vi "关键字子集.vi"(8 "图形程序":refnum<vi>, 9 "关键字":refnum<vi>, 10 "结束坐标":T1, 11 "起始坐标":T1) -> (0 "选中子集":cluster{"行":i32, "列":i32}[](array[cluster]))   [LabVIEW 2020]
uses:
  <vilib>/Utility/miscctls.llb/LVPoint32TypeDef.ctl
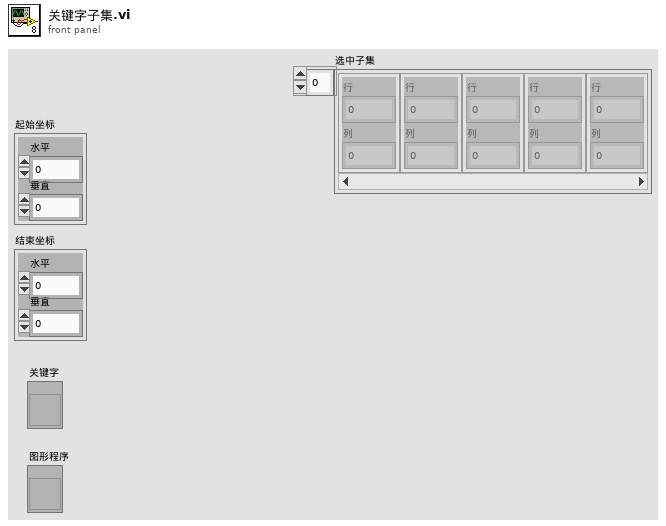
[diagram p1: front panel]
types:
  T1 = typedef "LVPoint32TypeDef.ctl" = cluster{"Horizontal":i32, "Vertical":i32}
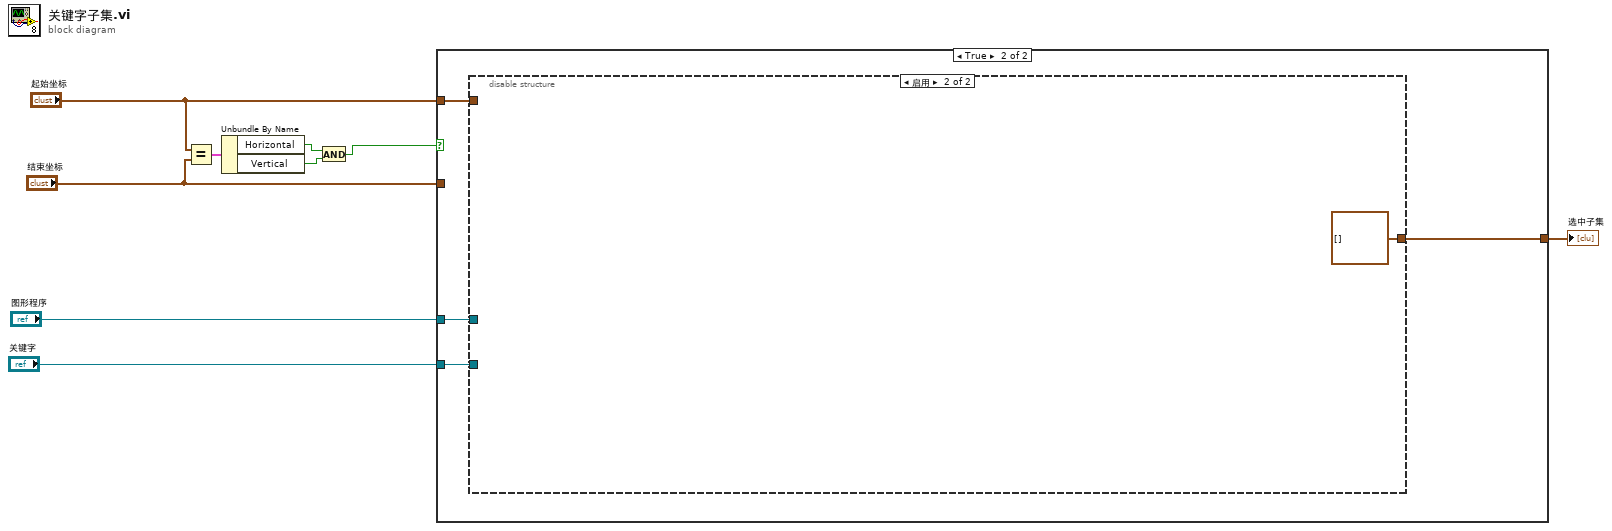
[diagram p0: block diagram]
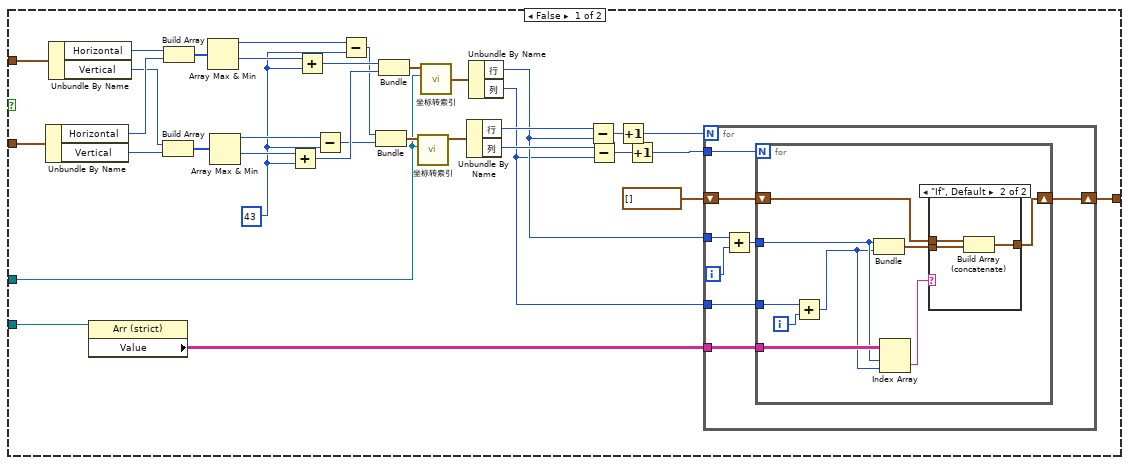
[diagram p2: hidden frame]
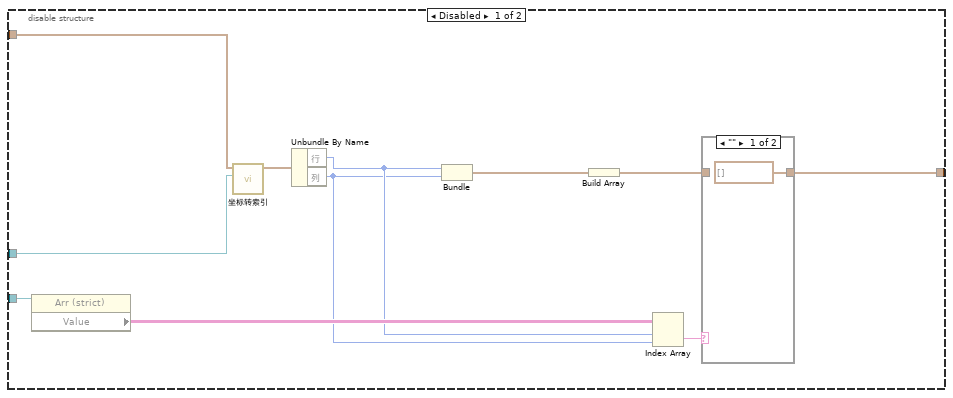
[diagram p4: hidden frame]
diagram:
  n1 = Equal?(x="起始坐标", y="结束坐标") -> (x = y?=w4:cluster{"Horizontal":bool, "Vertical":bool})
  n2 = Unbundle By Name(w4) -> ("Horizontal"=w3:bool, "Vertical"=w2:bool)
  n3 = And(x=w3, y=w2) -> (x .and. y?=w1:bool)
  n4 = case shown="True" w1 {
    tunnel: [w37 w66] -> w9
    tunnel: "起始坐标" -> [w34 w68]
    tunnel: "结束坐标" -> [w33 _]
    tunnel: "图形程序" -> [w11 w67]
    tunnel: "关键字" -> [w10 w65]
    frame False {
      w15 = 43 ("y")
      n5 = Unbundle By Name(w33) -> ("Horizontal"=w42:i32, "Vertical"=w40:i32)
      n6 = Unbundle By Name(w34) -> ("Horizontal"=w43:i32, "Vertical"=w41:i32)
      n7 = property class="Arr (strict)"(reference=w10) -> ("Value"=w35:string[][])  [unwired: 1 in, 2 out]
      n8 = Build Array(w41, w40) -> (w38:i32[])
      n9 = Build Array(w43, w42) -> (w39:i32[])
      n10 = Array Max & Min(array=w39) -> (max value=w32:i32, min value=w31:i32)  [unwired: 2 out]
      n11 = Array Max & Min(array=w38) -> (max value=w30:i32, min value=w29:i32)  [unwired: 2 out]
      n12 = Add(x=w29, y=w15) -> (x+y=w27:i32)
      n13 = Add(x=w31, y=w15) -> (x+y=w28:i32)
      n14 = Subtract(x=w30, y=w15) -> (x-y=w25:i32)
      n15 = Subtract(x=w32, y=w15) -> (x-y=w26:i32)
      n16 = Bundle(w26, w25) -> (w23:cluster{i32, i32})  [unwired: 1 in]
      n17 = Bundle(w28, w27) -> (w24:cluster{i32, i32})  [unwired: 1 in]
      n18 = call "坐标转索引.vi"("图形程序"=w11, "坐标"=w23) -> ("索引"=w21:cluster{"列":i32, "行":i32})  [unwired: 9 in]
      n19 = call "坐标转索引.vi"("图形程序"=w11, "坐标"=w24) -> ("索引"=w22:cluster{"列":i32, "行":i32})  [unwired: 9 in]
      n20 = Unbundle By Name(w21) -> ("行"=w20:i32, "列"=w19:i32)
      n21 = Unbundle By Name(w22) -> ("行"=w18:i32, "列"=w12:i32)
      n22 = Subtract(x=w20, y=w18) -> (x-y=w17:i32)
      n23 = Subtract(x=w19, y=w12) -> (x-y=w16:i32)
      n24 = Increment(x=w17) -> (x+1=w14:i32)
      n25 = Increment(x=w16) -> (x+1=w13:i32)
      n26 = for {
        N: w14 -> [_]
        tunnel: w18 -> [w51]
        tunnel: w12 -> [w48]
        shift-right: [w47] -> w37
        shift-left: cluster{i32, i32}[] [] -> [w46]
        tunnel: w35 -> [w45]
        tunnel: w13 -> [w44]
        i -> [w50]
        n27 = Add(x=w51, y=w50) -> (x+y=w49:i32)
        n28 = for {
          N: w44 -> [_]
          tunnel: w49 -> [w54]
          tunnel: w48 -> [w59]
          shift-right: [w57] -> w47
          shift-left: w46 -> [w56]
          tunnel: w45 -> [w55]
          i -> [w58]
          n29 = Add(x=w59, y=w58) -> (x+y=w53:i32)
          n30 = Bundle(w54, w53) -> (w60:cluster{i32, i32})  [unwired: 1 in]
          n31 = Index Array(array=w55, index (row)=w54, index (col)=w53) -> (element=w52:string)
          n32 = case shown="\"If\", Default" w52 {
            tunnel: w60 -> [_ w64]
            tunnel: [w61 w63] -> w57
            tunnel: w56 -> [w61 w62]
            frame "" {
            }
            frame "If", Default {
              n33 = Build Array (concatenate)(w62, w64) -> (w63:cluster{i32, i32}[])
            }
          }
        }
      }
    }
    frame True {
      n34 = disable-structure shown="启用" {
        disable-tunnel: w68 -> [w79 _]
        disable-tunnel: w67 -> [w78 _]
        disable-tunnel: [w74 cluster{"行":i32, "列":i32}[] []] -> w66
        disable-tunnel: w65 -> [w72 _]
        frame Disabled {
          n35 = property class="Arr (strict)"(reference=w72) -> ("Value"=w71:string[][])  [unwired: 1 in, 2 out]
          n36 = call "坐标转索引.vi"("图形程序"=w78, "坐标"=w79) -> ("索引"=w77:cluster{"列":i32, "行":i32})  [unwired: 9 in]
          n37 = Unbundle By Name(w77) -> ("行"=w70:i32, "列"=w69:i32)
          n38 = Bundle("行"=w70, "列"=w69) -> (w76:cluster{"行":i32, "列":i32})  [unwired: 1 in]
          n39 = Build Array(w76) -> (w75:cluster{"行":i32, "列":i32}[])
          n40 = Index Array(array=w71, index (row)=w70, index (col)=w69) -> (element=w73:string)
          n41 = case shown="\"\"" w73 {
            tunnel: w75 -> [_ w81]
            tunnel: [cluster{i32, i32}[] [] w81] -> w74
            frame "" {
            }
            frame "If", Default {
            }
          }
        }
        frame Enabled {
        }
      }
    }
  }
  "选中子集" <- w9
